vi "总磷总氮备用系数读取.vi"(8 "error in (no error)":errorcluster caption="错误输入（无错误）", 11 "测量参数":enum16{"总磷", "总氮"}(ring)) -> (0 "error out":errorcluster caption="错误输出", 3 "备用系数":T1)   [LabVIEW 2016, in "斯坦道仪器.lvlib"]
panel:
  in  "测量模式":enum16{"水样测量", "空白核查", "跨度核查", "标样核查", "加标回收"}(ring)
  in  "量程":enum16{"低量程", "高量程"}(ring)
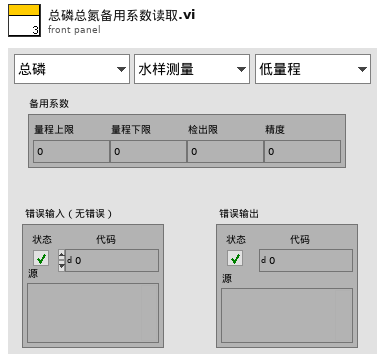
[diagram p1: front panel]
types:
  T1 = cluster{"量程上限":dbl, "量程下限":dbl, "检出限":dbl, "精度":dbl}
  T2 = cluster{"数组[0]":dbl, "数组[1]":dbl, "数组[2]":dbl, "数组[3]":dbl}
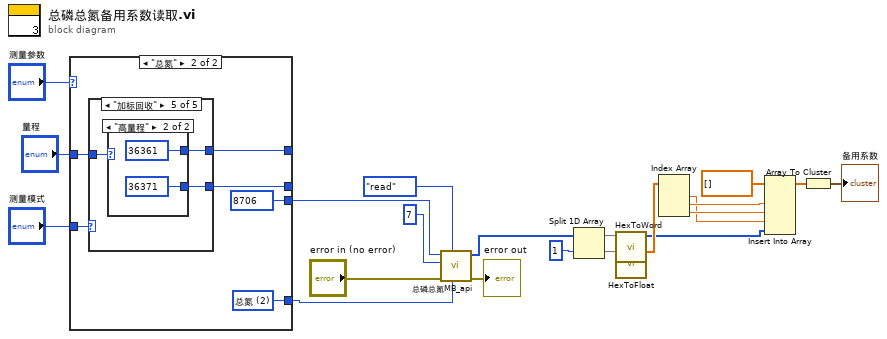
[diagram p0: block diagram]
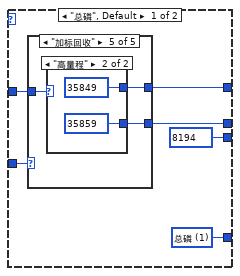
[diagram p2: hidden frame]
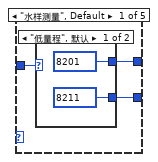
[diagram p3: hidden frame]
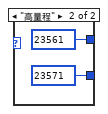
[diagram p4: hidden frame]
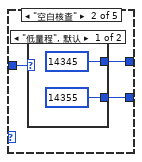
[diagram p5: hidden frame]
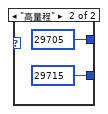
[diagram p6: hidden frame]
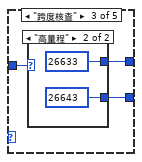
[diagram p7: hidden frame]
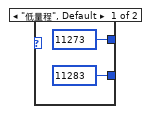
[diagram p8: hidden frame]
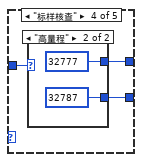
[diagram p9: hidden frame]
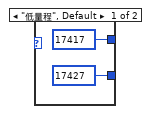
[diagram p10: hidden frame]
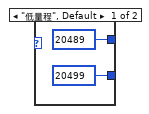
[diagram p11: hidden frame]
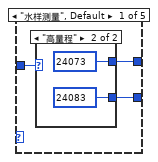
[diagram p12: hidden frame]
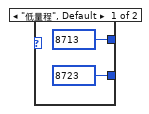
[diagram p13: hidden frame]
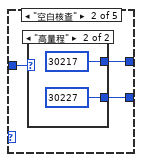
[diagram p14: hidden frame]
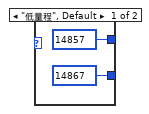
[diagram p15: hidden frame]
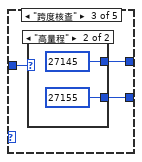
[diagram p16: hidden frame]
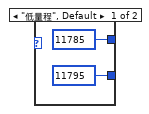
[diagram p17: hidden frame]
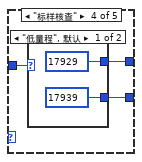
[diagram p18: hidden frame]
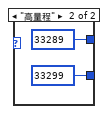
[diagram p19: hidden frame]
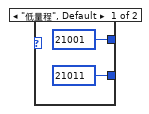
[diagram p20: hidden frame]
diagram:
  n1 = case shown="\"总氮\"" "测量参数" {
    tunnel: "测量模式" -> [w27 w65]
    tunnel: "量程" -> [w26 w66]
    tunnel: [w25 w68] -> w2
    tunnel: [w24 w63] -> _
    tunnel: [w23 w64] -> _
    tunnel: [u16 8194 ("starting address") u16 8706 ("starting address")] -> w17
    frame "总磷", Default {
      w25 = u16 1 items=["总磷"=1, "氨氮"=3] ("站号")
      n2 = case shown="\"加标回收\"" w27 {
        tunnel: w26 -> [w30 w37 w44 w51 w58]
        tunnel: [w29 w36 w43 w50 w57] -> w24
        tunnel: [w28 w35 w42 w49 w56] -> w23
        frame "水样测量", Default {
          n3 = case shown="\"低量程\", 默认" w30 {
            tunnel: [u16 8211 ("starting address") u16 23571 ("starting address")] -> w29
            tunnel: [u16 8201 ("starting address") u16 23561 ("starting address")] -> w28
            frame "低量程", Default {
            }
            frame "高量程" {
            }
          }
        }
        frame "空白核查" {
          n4 = case shown="\"低量程\", 默认" w37 {
            tunnel: [u16 14355 ("starting address") u16 29715 ("starting address")] -> w36
            tunnel: [u16 14345 ("starting address") u16 29705 ("starting address")] -> w35
            frame "低量程", Default {
            }
            frame "高量程" {
            }
          }
        }
        frame "跨度核查" {
          n5 = case shown="\"高量程\"" w44 {
            tunnel: [u16 11283 ("starting address") u16 26643 ("starting address")] -> w43
            tunnel: [u16 11273 ("starting address") u16 26633 ("starting address")] -> w42
            frame "低量程", Default {
            }
            frame "高量程" {
            }
          }
        }
        frame "标样核查" {
          n6 = case shown="\"高量程\"" w51 {
            tunnel: [u16 17427 ("starting address") u16 32787 ("starting address")] -> w50
            tunnel: [u16 17417 ("starting address") u16 32777 ("starting address")] -> w49
            frame "低量程", Default {
            }
            frame "高量程" {
            }
          }
        }
        frame "加标回收" {
          n7 = case shown="\"高量程\"" w58 {
            tunnel: [u16 20499 ("starting address") u16 35859 ("starting address")] -> w57
            tunnel: [u16 20489 ("starting address") u16 35849 ("starting address")] -> w56
            frame "低量程", Default {
            }
            frame "高量程" {
            }
          }
        }
      }
    }
    frame "总氮" {
      w68 = u16 2 items=["总磷"=1, "总氮"=2, "氨氮"=3] ("站号")
      n8 = case shown="\"加标回收\"" w65 {
        tunnel: w66 -> [w71 w78 w85 w92 w99]
        tunnel: [w70 w77 w84 w91 w98] -> w63
        tunnel: [w69 w76 w83 w90 w97] -> w64
        frame "水样测量", Default {
          n9 = case shown="\"高量程\"" w71 {
            tunnel: [u16 8723 ("starting address") u16 24083 ("starting address")] -> w70
            tunnel: [u16 8713 ("starting address") u16 24073 ("starting address")] -> w69
            frame "低量程", Default {
            }
            frame "高量程" {
            }
          }
        }
        frame "空白核查" {
          n10 = case shown="\"高量程\"" w78 {
            tunnel: [u16 14867 ("starting address") u16 30227 ("starting address")] -> w77
            tunnel: [u16 14857 ("starting address") u16 30217 ("starting address")] -> w76
            frame "低量程", Default {
            }
            frame "高量程" {
            }
          }
        }
        frame "跨度核查" {
          n11 = case shown="\"高量程\"" w85 {
            tunnel: [u16 11795 ("starting address") u16 27155 ("starting address")] -> w84
            tunnel: [u16 11785 ("starting address") u16 27145 ("starting address")] -> w83
            frame "低量程", Default {
            }
            frame "高量程" {
            }
          }
        }
        frame "标样核查" {
          n12 = case shown="\"低量程\", 默认" w92 {
            tunnel: [u16 17939 ("starting address") u16 33299 ("starting address")] -> w91
            tunnel: [u16 17929 ("starting address") u16 33289 ("starting address")] -> w90
            frame "低量程", Default {
            }
            frame "高量程" {
            }
          }
        }
        frame "加标回收" {
          n13 = case shown="\"高量程\"" w99 {
            tunnel: [u16 21011 ("starting address") u16 36371 ("starting address")] -> w98
            tunnel: [u16 21001 ("starting address") u16 36361 ("starting address")] -> w97
            frame "低量程", Default {
            }
            frame "高量程" {
            }
          }
        }
      }
    }
  }
  n14 = call "总磷总氮MB_api.vi"("Slave ID"=w2, "STEP"=enum16{"open", "read", "write", "close"}."read", "Error in"="error in (no error)", "quantity"=u16 7, "starting address"=w17) -> ("error out"=→"error out":errorcluster, "Registers"=w14:u16[])  [unwired: 3 in, 2 out]
  n15 = Split 1D Array(array=w14, index=1 ("索引")) -> (first subarray=w12:u16[], second subarray=w11:u16[])
  n16 = call "HexToWord.vi"("数组"=w12) -> ("WORD"=w4:u16[])  [unwired: 10 in]
  n17 = call "HexToFloat.vi"("数组"=w11) -> ("FLOAT"=w9:sgl[])  [unwired: 10 in]
  n18 = Index Array(array=w9) -> (element #1=w5:sgl, element #2=w7:sgl, element #3=w6:sgl)  [unwired: 3 in]
  n19 = Insert Into Array(array=dbl[] [] ("数组"), new element #1=w7, new element #2=w6, new element #3=w5, new element #4=w4) -> (w3:dbl[])  [unwired: 1 in]
  n20 = Array To Cluster(array=w3) -> (cluster=→"备用系数":T2)
